vi "Split NIC Config Groups.vi"(11 "Network Interface Config":string) -> (3 "NIC Config Groups":string[](array[string]))   [LabVIEW 2019, in "LMH-LINX.lvlib"]
uses:
  <vilib>/MakerHub/LINX/LMH-LINX.lvlib
  <vilib>/regexp/Match Regular Expression.xnode
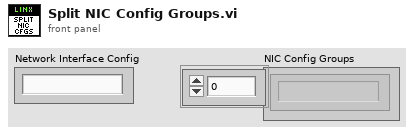
[diagram p1: front panel]
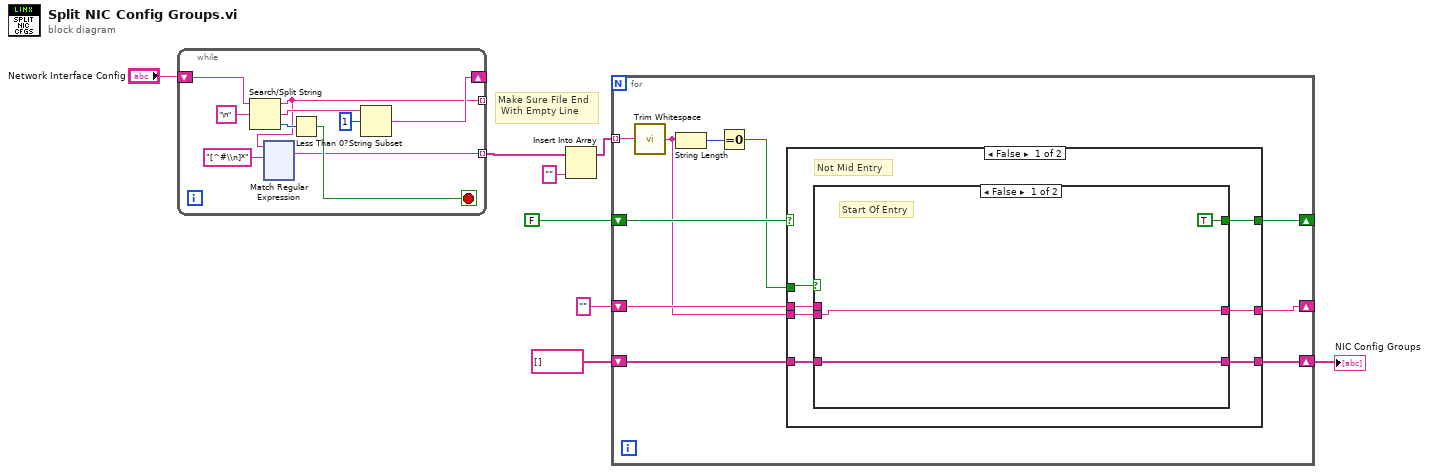
[diagram p0: block diagram]
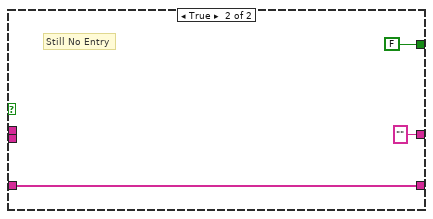
[diagram p2: hidden frame]
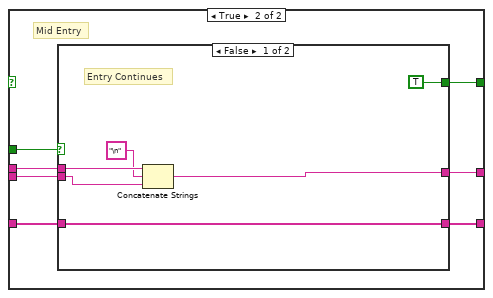
[diagram p3: hidden frame]
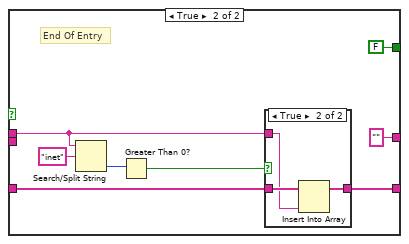
[diagram p4: hidden frame]
diagram:
  # "Make Sure File End\n With Empty Line"
  n1 = while {
    tunnel: [w10] -> _ mode=indexing
    shift-right: [w12] -> _
    shift-left: "Network Interface Config" -> [w15]
    tunnel: [w9] -> w6 mode=indexing
    stop <- w16 stop-if-true
    n2 = Search/Split String(string=w15, search string/char (-)="\n") -> (substring before match=w10:string, match + rest of string=w14:string, offset of match=w17:i32)  [unwired: 1 in]
    n3 = xnode "Match Regular Expression"("input string"=w10, "regular expression"="[^#\\n]*") -> ("whole match"=w9:string)  [unwired: 4 in, 4 out]
    n4 = Less Than 0?(x=w17) -> (x < 0?=w16:bool)
    n5 = String Subset(string=w14, offset (0)=1) -> (substring=w12:string)  [unwired: 1 in]
  }
  n6 = Insert Into Array(array=w6, new element="" ("new element/subarray")) -> (w7:string[])  [unwired: 1 in]
  n7 = for {
    tunnel: w7 -> [w139] mode=indexing
    shift-right: [w135] -> _
    shift-left: FALSE -> [w137]
    shift-right: [w132] -> _
    shift-left: "" -> [w134]
    shift-right: [w130] -> w5
    shift-left: string[] [] -> [w131]
    n8 = call <vilib>:"Trim Whitespace.vi"("string"=w139) -> ("trimmed string"=w133:string)  [unwired: 1 in]
    n9 = String Length(string=w133) -> (length=w138:i32)
    n10 = Equal To 0?(x=w138) -> (x = 0?=w136:bool)
    n11 = case shown="False" w137 {
      tunnel: w136 -> [w146 w159]
      tunnel: [w145 w158] -> w135
      tunnel: w134 -> [w144 w157]
      tunnel: w133 -> [w143 w156]
      tunnel: [w142 w155] -> w132
      tunnel: w131 -> [w140 w154]
      tunnel: [w141 w153] -> w130
      frame False {
        # "Not Mid Entry"
        n12 = case shown="False" w146 {
          tunnel: [TRUE FALSE] -> w145
          tunnel: w144 -> [_ _]
          tunnel: w143 -> [w148 _]
          tunnel: [w148 ""] -> w142
          tunnel: [w147 w150] -> w141
          tunnel: w140 -> [w147 w150]
          frame False {
            # "Start Of Entry"
          }
          frame True {
            # "Still No Entry"
          }
        }
      }
      frame True {
        # "Mid Entry"
        n13 = case shown="False" w159 {
          tunnel: [TRUE FALSE] -> w158
          tunnel: w157 -> [w164 w169]
          tunnel: w156 -> [w161 _]
          tunnel: [w163 ""] -> w155
          tunnel: w154 -> [w162 w172]
          tunnel: [w162 w171] -> w153
          frame False {
            # "Entry Continues"
            n14 = Concatenate Strings(w164, "\n" ("search string/char (-)"), w161) -> (w163:string)
          }
          frame True {
            # "End Of Entry"
            n15 = Search/Split String(string=w169, search string/char (-)="inet") -> (offset of match=w167:i32)  [unwired: 1 in, 2 out]
            n16 = Greater Than 0?(x=w167) -> (x > 0?=w166:bool)
            n17 = case shown="True" w166 {
              tunnel: w172 -> [w174 w177]
              tunnel: [w174 w176] -> w171
              tunnel: w169 -> [_ w175]
              frame False {
              }
              frame True {
                n18 = Insert Into Array(array=w177, new element=w175) -> (w176:string[])  [unwired: 1 in]
              }
            }
          }
        }
      }
    }
  }
  "NIC Config Groups" <- w5
